vi "If AND Then Else.vi"(7 "AND Condition":bool, 8 "AND Conditional Text":string, 9 "Current Text":string) -> (3 "Current Text Out":string)   [LabVIEW 2010]
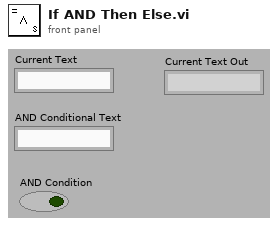
[diagram p1: front panel]
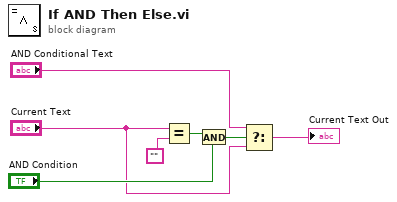
[diagram p0: block diagram]
diagram:
  n1 = Equal?(x="Current Text", y="") -> (x = y?=w3:bool)
  n2 = And(x=w3, y="AND Condition") -> (x .and. y?=w5:bool)
  n3 = Select(t="AND Conditional Text", s=w5, f="Current Text") -> (s? t:f=→"Current Text Out":string)
